vi "Init.vi"(8 "error in (no error)":errorcluster, 11 "HSL-2000 in":refnum<class "HSL-2000.lvclass">) -> (0 "error out":errorcluster, 3 "HSL-2000 out":refnum<class "HSL-2000.lvclass">)   [LabVIEW 2014, in "HSL-2000.lvclass"]
uses:
  HSL-2000.lvclass
  Santec.lvclass
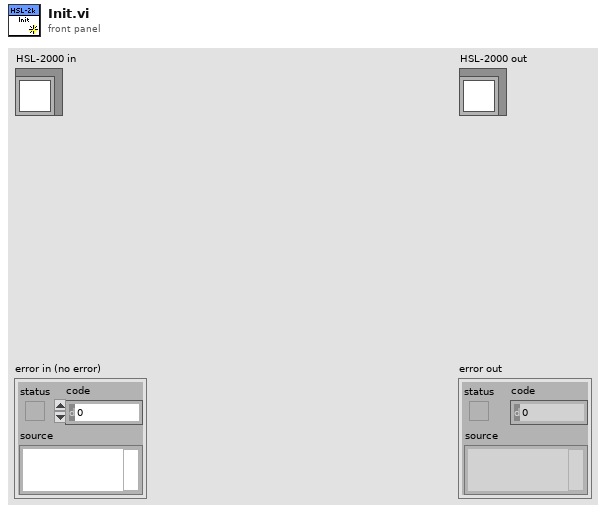
[diagram p1: front panel]
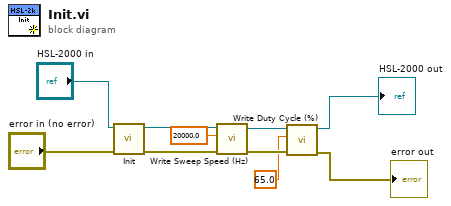
[diagram p0: block diagram]
diagram:
  n1 = call-parent "Init.vi"("error in (no error)"="error in (no error)", "Santec in"="HSL-2000 in") -> ("error out"=w7:errorcluster, "Santec out"=w8:refnum<class "HSL-2000.lvclass">)  [unwired: 8 in]
  n2 = call-dynamic "Write Sweep Speed (Hz).vi"("error in (no error)"=w7, "Sweep Speed (Hz)"=20000.0, "Laser in"=w8) -> ("error out"=w5:errorcluster, "Laser out"=w4:refnum<class "HSL-2000.lvclass">)  [unwired: 7 in]
  n3 = call-dynamic "Write Duty Cycle (%).vi"("error in (no error)"=w5, "Duty Cycle (%)"=65.0, "Laser in"=w4) -> ("error out"=→"error out":errorcluster, "Laser out"=→"HSL-2000 out":refnum<class "HSL-2000.lvclass">)  [unwired: 7 in]
